vi "Stream from HS PGcamera.vi"(2 "External Stop":refnum<vi>) -> ()   [LabVIEW 2019]
uses:
  <vilib>/userdefined/High Color/IMAQdx.ctl
  <vilib>/vision/driver/NI_Vision_Acquisition_Software.lvlib
  <resource>/objmgr/imaqdx.rc
panel:
  in  "Session In":T1="cam0"
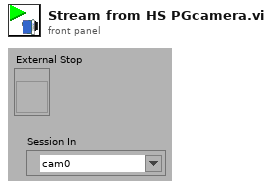
[diagram p1: front panel]
types:
  T1 = typedef "IMAQdx.ctl" = refnum<k21>
  T2 = typedef "IMAQ Image.ctl" = refnum<image>
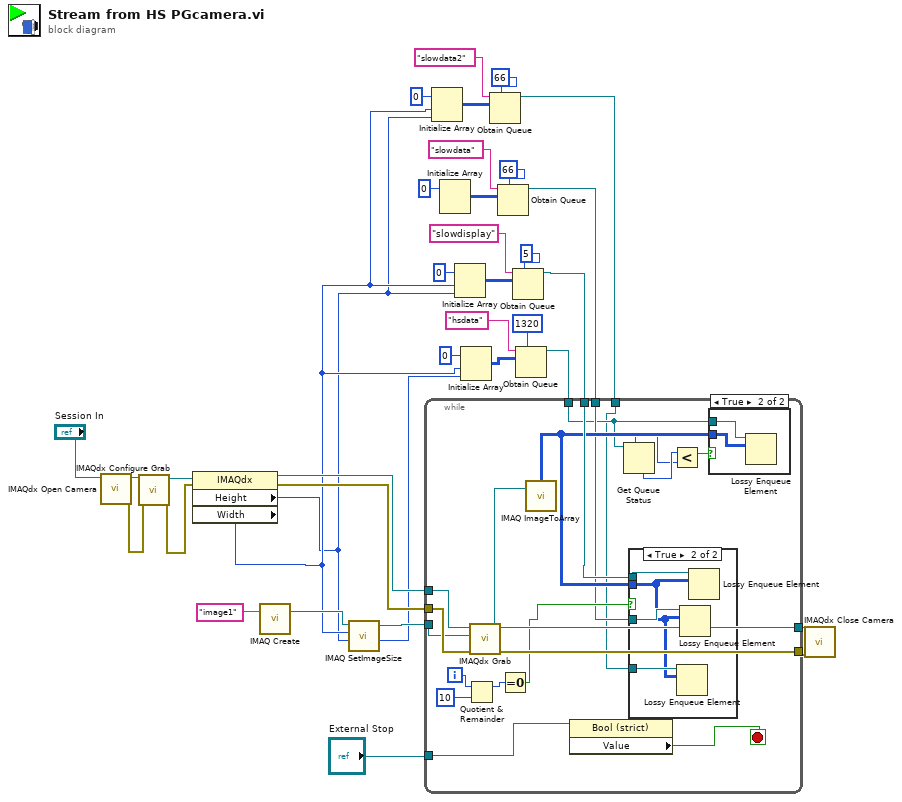
[diagram p0: block diagram]
diagram:
  n1 = call <vilib>:"IMAQdx Open Camera.vi"("Session In"="Session In") -> ("error out"=w20:errorcluster, "Session Out"=w21:T1)  [unwired: 9 in]
  n2 = call <vilib>:"IMAQdx Configure Grab.vi"("error in"=w20, "Session In"=w21) -> ("error out"=w17:errorcluster, "Session Out"=w18:T1)  [unwired: 8 in]
  n3 = property class="IMAQdx"(reference=w18, error in=w17) -> (reference out=w16:T1, error out=w15:errorcluster, "Height"=w1:u32, "Width"=w2:u32)
  n4 = call "IMAQ Create"("Image Name"="image1") -> ("New Image"=w35:T2)  [unwired: 4 in, 1 out]
  n5 = call "IMAQ SetImageSize"("Y Resolution"=w1, "X Resolution"=w2, "Image"=w35) -> ("Image Out"=w34:T2)  [unwired: 2 in, 1 out]
  n6 = Initialize Array(i16 0 ("element"), w2, w1) -> (w4:i16[][])
  n7 = Initialize Array(i16 0 ("element")) -> (w9:i16[][])  [unwired: 2 in]
  n8 = Initialize Array(u8 0 ("element"), w2, w1) -> (w22:u8[][])
  n9 = Initialize Array(u8 0 ("element"), w2, w1) -> (w27:u8[][])
  n10 = Obtain Queue(max queue size (-1, unlimited)=66, name (unnamed)="slowdata2", element data type=w4) -> (queue out=w3:refnum<queue>)  [unwired: 2 in, 2 out]
  n11 = Obtain Queue(max queue size (-1, unlimited)=66, name (unnamed)="slowdata", element data type=w9) -> (queue out=w8:refnum<queue>)  [unwired: 2 in, 2 out]
  n12 = Obtain Queue(max queue size (-1, unlimited)=5, name (unnamed)="slowdisplay", element data type=w22) -> (queue out=w26:refnum<queue>)  [unwired: 2 in, 2 out]
  n13 = Obtain Queue(max queue size (-1, unlimited)=1320, name (unnamed)="hsdata", element data type=w27) -> (queue out=w33:refnum<queue>)  [unwired: 2 in, 2 out]
  n14 = while {
    tunnel: w34 -> [w51]
    tunnel: w33 -> [w40]
    tunnel: "External Stop" -> [w54]
    tunnel: w26 -> [w43]
    tunnel: w16 -> [w53]
    tunnel: w15 -> [w52]
    tunnel: [w49] -> w14
    tunnel: [w48] -> w13
    tunnel: w8 -> [w41]
    tunnel: w3 -> [w36]
    i -> [w47]
    stop <- w55 stop-if-true
    n15 = Quotient & Remainder(x=w47, y=10) -> (x-y*floor(x/y)=w45:i32)  [unwired: 1 out]
    n16 = call <vilib>:"IMAQdx Grab.vi"("error in"=w52, "Image In"=w51, "Session In"=w53) -> ("error out"=w48:errorcluster, "Image Out"=w50:T2, "Session Out"=w49:T1)  [unwired: 5 in, 1 out]
    n17 = Equal To 0?(x=w45) -> (x = 0?=w44:bool)
    n18 = call "IMAQ ImageToArray"("Image"=w50) -> ("Image Pixels (U8)"=w42:u8[][])  [unwired: 3 in, 4 out]
    n19 = property class="Bool (strict)"(reference=w54) -> ("Value"=w55:bool)  [unwired: 1 in, 2 out]
    n20 = Get Queue Status(queue=w40) -> (max queue size=w38:i32, # elements in queue=w39:i32)  [unwired: 2 in, 6 out]
    n21 = case shown="True" w44 {
      tunnel: w43 -> [_ w61]
      tunnel: w42 -> [_ w58]
      tunnel: w41 -> [_ w60]
      tunnel: w36 -> [_ w59]
      frame False {
      }
      frame True {
        n22 = Lossy Enqueue Element(queue=w59, element=w58) -> ()  [unwired: 1 in, 4 out]
        n23 = Lossy Enqueue Element(queue=w60, element=w58) -> ()  [unwired: 1 in, 4 out]
        n24 = Lossy Enqueue Element(queue=w61, element=w58) -> ()  [unwired: 1 in, 4 out]
      }
    }
    n25 = Less?(x=w39, y=w38) -> (x < y?=w37:bool)
    n26 = case shown="True" w37 {
      tunnel: w42 -> [_ w56]
      tunnel: w40 -> [_ w57]
      frame False {
      }
      frame True {
        n27 = Lossy Enqueue Element(queue=w57, element=w56) -> ()  [unwired: 1 in, 4 out]
      }
    }
  }
  n28 = call <vilib>:"IMAQdx Close Camera.vi"("error in"=w13, "Session In"=w14) -> ()  [unwired: 9 in, 1 out]
